vi "PrepareUIShadow.vi"(8 "error in (no error)":errorcluster, 11 "Shadow in":refnum<class "Shadow.lvclass">) -> (0 "error out":errorcluster, 3 "Shadow out":refnum<class "Shadow.lvclass">)   [LabVIEW 2021, in "UIShadow.lvlib" / "Shadow.lvclass"]
uses:
  Shadow.lvclass
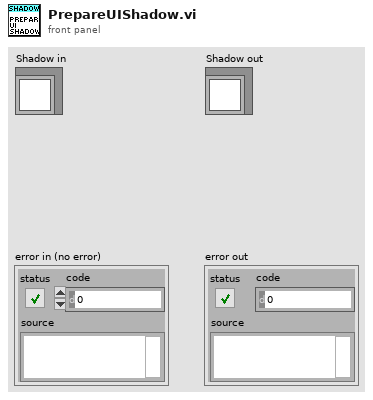
[diagram p1: front panel]
types:
  T1 = enum32{"Invalid", "Standard", "Closed", "Hidden", "Minimized", "Maximized"}
  T2 = typedef "UIShadow.lvlib/Shadow.lvclass/Data.ctl" = cluster{"VI Refnum":refnum<vi>, "ShadowColor":u32, "Offset":i16, "Transparancy":i32, "UIShadowRef":refnum<vi>, "Activate?":bool}
  T3 = enum32{"Invalid", "Default", "Floating", "Floating/Auto-Hide", "Modal"}
  T4 = typedef "LVRectTypeDef.ctl" = cluster{"Left":i16, "Top":i16, "Right":i16, "Bottom":i16}
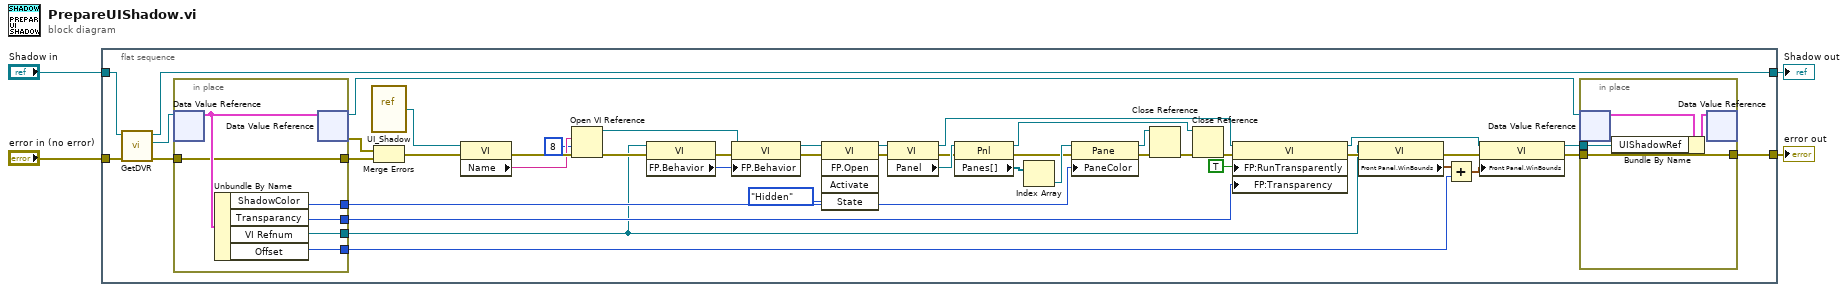
[diagram p0: block diagram]
diagram:
  n1 = flat-sequence {
    tunnel: "Shadow in" -> [w39]
    tunnel: [w40] -> w2
    tunnel: [w13] -> w4
    tunnel: "error in (no error)" -> [w41]
    frame #0 {
      n2 = call "GetDVR.vi"("error in (no error)"=w41, "Shadow in"=w39) -> ("error out"=w38:errorcluster, "DVR"=w37:refnum<data-value>, "Shadow out"=w40:refnum<class "Shadow.lvclass">)  [unwired: 7 in]
      n3 = in-place {
        in-place-border: w38 -> [w51]
        in-place-border: [w55] -> w7
        in-place-border: [w54] -> w36
        in-place-border: [w53] -> w34
        in-place-border: [w52] -> w27
        in-place-border: [w51] -> w19
        n4 = in-place-dvr #1(w37) -> (w56:T2)  [unwired: 1 out]
        n5 = Unbundle By Name(w56) -> ("ShadowColor"=w52:u32, "Transparancy"=w54:i32, "VI Refnum"=w55:refnum<vi>, "Offset"=w53:i16)
        n6 = in-place-dvr #1(w56) -> (w15:refnum<data-value>, w17:errorcluster)
      }
      n7 = vi-ref "UI_Shadow.vi"() -> (w33:refnum<vi>)
      n8 = Merge Errors(w17, w19) -> (w18:errorcluster)
      n9 = property class="VI"(reference=w33, error in=w18) -> (error out=w48:errorcluster, "Name"=w45:string)  [unwired: 1 out]
      n10 = Open VI Reference(vi path=w45, options=8, error in (no error)=w48) -> (vi reference=w11:refnum<vi>, error out=w9:errorcluster)  [unwired: 3 in]
      n11 = property class="VI"(reference=w7, error in=w9) -> (error out=w8:errorcluster, "FP.Behavior"=w6:T3)  [unwired: 1 out]
      n12 = property class="VI"(reference=w11, error in=w8, "FP.Behavior"=w6) -> (reference out=w10:refnum<vi>, error out=w12:errorcluster)
      n13 = invoke class="VI" method="FP.Open"(reference=w10, error in=w12, "State"=T1."Hidden") -> (reference out=w32:refnum<vi>, error out=w49:errorcluster)  [unwired: 2 in, 3 out]
      n14 = property class="VI"(reference=w32, error in=w49) -> (reference out=w31:refnum<vi>, error out=w21:errorcluster, "Panel"=w30:refnum<vi>)
      n15 = property class="Pnl"(reference=w30, error in=w21) -> (reference out=w24:refnum<vi>, error out=w20:errorcluster, "Panes[]"=w29:refnum<vi>[])
      n16 = Index Array(array=w29) -> (element=w28:refnum<vi>)  [unwired: 1 in]
      n17 = property class="Pane"(reference=w28, error in=w20, "PaneColor"=w27) -> (reference out=w25:refnum<vi>, error out=w26:errorcluster)
      n18 = Close Reference(reference=w25, error in (no error)=w26) -> (error out=w23:errorcluster)
      n19 = Close Reference(reference=w24, error in (no error)=w23) -> (error out=w22:errorcluster)
      n20 = property class="VI"(reference=w31, error in=w22, "FP:RunTransparently"=TRUE ("Front Panel Window:Run VI Transparently"), "FP:Transparency"=w36) -> (reference out=w46:refnum<vi>, error out=w43:errorcluster)
      n21 = property class="VI"(reference=w7, error in=w43) -> (error out=w42:errorcluster, "Front Panel.WinBounds"=w44:T4)  [unwired: 1 out]
      n22 = Add(x=w44, y=w34) -> (x+y=w35:T4)
      n23 = property class="VI"(reference=w46, error in=w42, "Front Panel.WinBounds"=w35) -> (reference out=w14:refnum<vi>, error out=w16:errorcluster)
      n24 = in-place {
        in-place-border: w16 -> [w57]
        in-place-border: w14 -> [w59]
        in-place-border: [w57] -> w13
        n25 = in-place-dvr #2(w15) -> (w60:T2)  [unwired: 1 out]
        n26 = Bundle By Name(cluster=w60, "UIShadowRef"=w59) -> (w58:T2)
        n27 = in-place-dvr #2(w58) -> ()  [unwired: 2 out]
      }
    }
  }
  "error out" <- w4
  "Shadow out" <- w2
